vi "Autonomous.vi"() -> ()   [LabVIEW 2019]
doc: "This VI starts when autonomous period begins, and will automatically be terminated when it ends. You can carry out timed or sensor driven operations directly to I/O or to subsystems without needing to return to the caller."
uses:
  <vilib>/Rock Robotics/WPI/Utilities/WPI_GetSetVariantRefNum.vi
  <vilib>/Rock Robotics/Network Tables/NT Read String.vi
panel:
  in  "goto":string
  in  "start":string
  in  "milliseconds to wait":u32
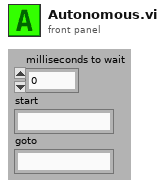
[diagram p1: front panel]
types:
  T1 = typedef "WPI_JoystickDevRef.ctl" = cluster{"Device":T2}
  T2 = typedef "WPI_JoystickDeviceEnum.ctl" = enum16{"USB 0", "USB 1", "USB 2", "USB 3", "USB 4", "USB 5"}
  T3 = typedef "Command Status Info.ctl" = cluster{"Name":string, "Status":T4, "notifier out":T5}
  T4 = typedef "Completion Status.ctl" = enum16{"Successful", "Aborted", "Incomplete"}
  T5 = typedef "Completion Notifier.ctl" = refnum<notifier>
  T6 = typedef "WPI_MotorControlDeviceRef.ctl" = cluster{"DeviceStatus":errorcluster, "Type":T7, "PWM":cluster{"PWM Channel":T8, "DeadBand":T9}, "CAN":cluster{"Device Number":u8, "SetOutput VI Ref":variant, "GetOutput VI Ref":variant, "Enable VI Ref":variant, "Disable VI Ref":variant, "Data":variant}, "Invert":bool, "DIO PWM":cluster{"PWM \"Enable\" Channel":T8, "DIOChannel":T10, "PWM Rate":dbl}}
  T7 = typedef "WPI_MotorControlType.ctl" = enum16{"PWM", "CAN", "DIO PWM"}
  T8 = typedef "FPGA_DIOPWMChannel.ctl" = enum8{"PWM 0", "PWM 1", "PWM 2", "PWM 3", "PWM 4", "PWM 5", "PWM 6", "PWM 7", "PWM 8", "PWM 9", "PWM MXP 0", "PWM MXP 1", "PWM MXP 2", "PWM MXP 3", "PWM MXP 4", "PWM MXP 5", "PWM MXP 6", "PWM MXP 7", "PWM MXP 8", "PWM MXP 9", "Invalid"}
  T9 = typedef "WPI_PWMDeadband.ctl" = cluster{"Name":string, "maxPositivePwm":i32, "minPositivePwm":i32, "centerPwm":i32, "maxNegativePwm":i32, "minNegativePwm":i32, "angularRange":u16}
  T10 = typedef "FPGA_DIOChannel.ctl" = enum8{"DIO 0", "DIO 1", "DIO 2", "DIO 3", "DIO 4", "DIO 5", "DIO 6", "DIO 7", "DIO 8", "DIO 9", "DIO MXP 0", "DIO MXP 1", "DIO MXP 2", "DIO MXP 3", "DIO MXP 4", "DIO MXP 5", "DIO MXP 6", "DIO MXP 7", "DIO MXP 8", "DIO MXP 9", "DIO MXP 10", "DIO MXP 11", "DIO MXP 12", "DIO MXP 13", "DIO MXP 14", "DIO MXP 15", "SPI Port CS1", "SPI Port CS2", "SPI Port CS3", "SPI Port MISO", "SPI Port MOSI", "Invalid"}
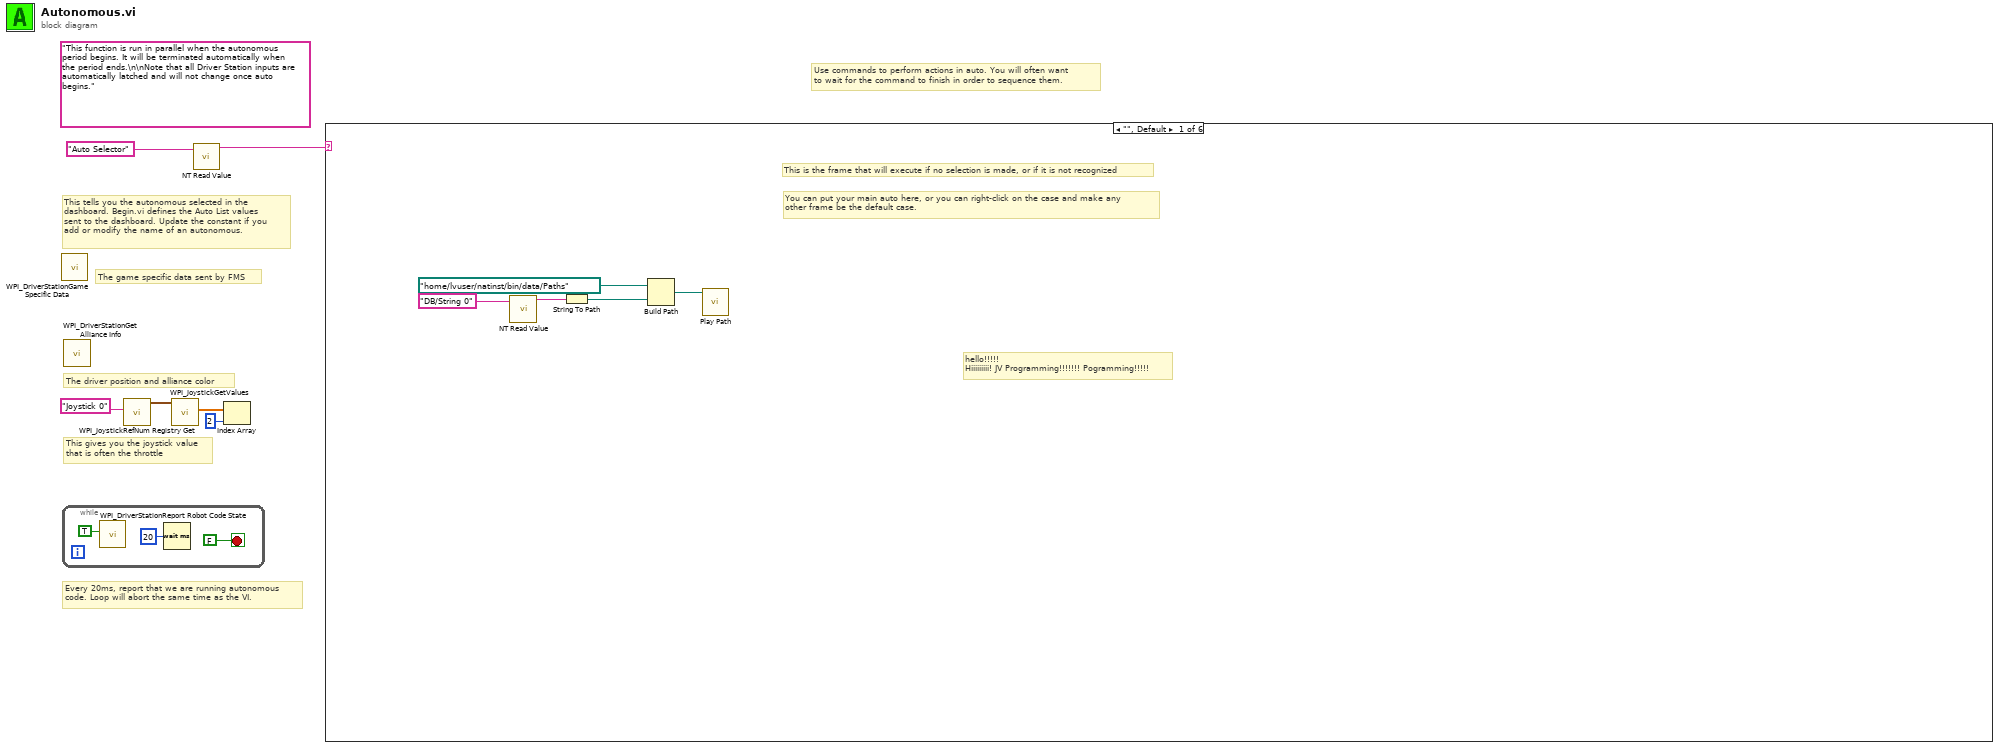
[diagram p0: block diagram]
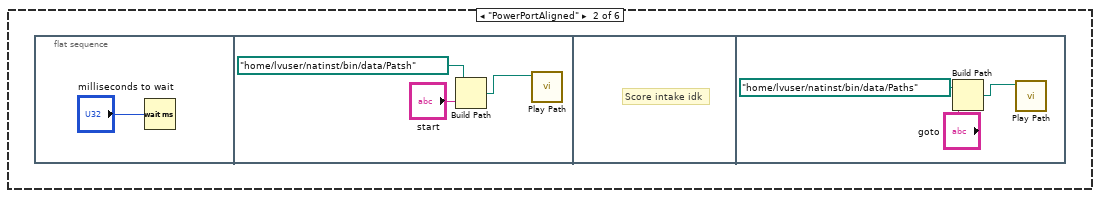
[diagram p2: hidden frame]
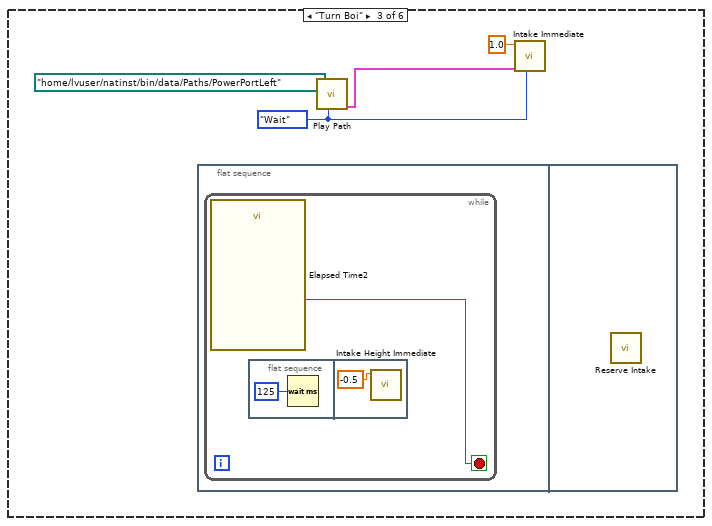
[diagram p3: hidden frame]
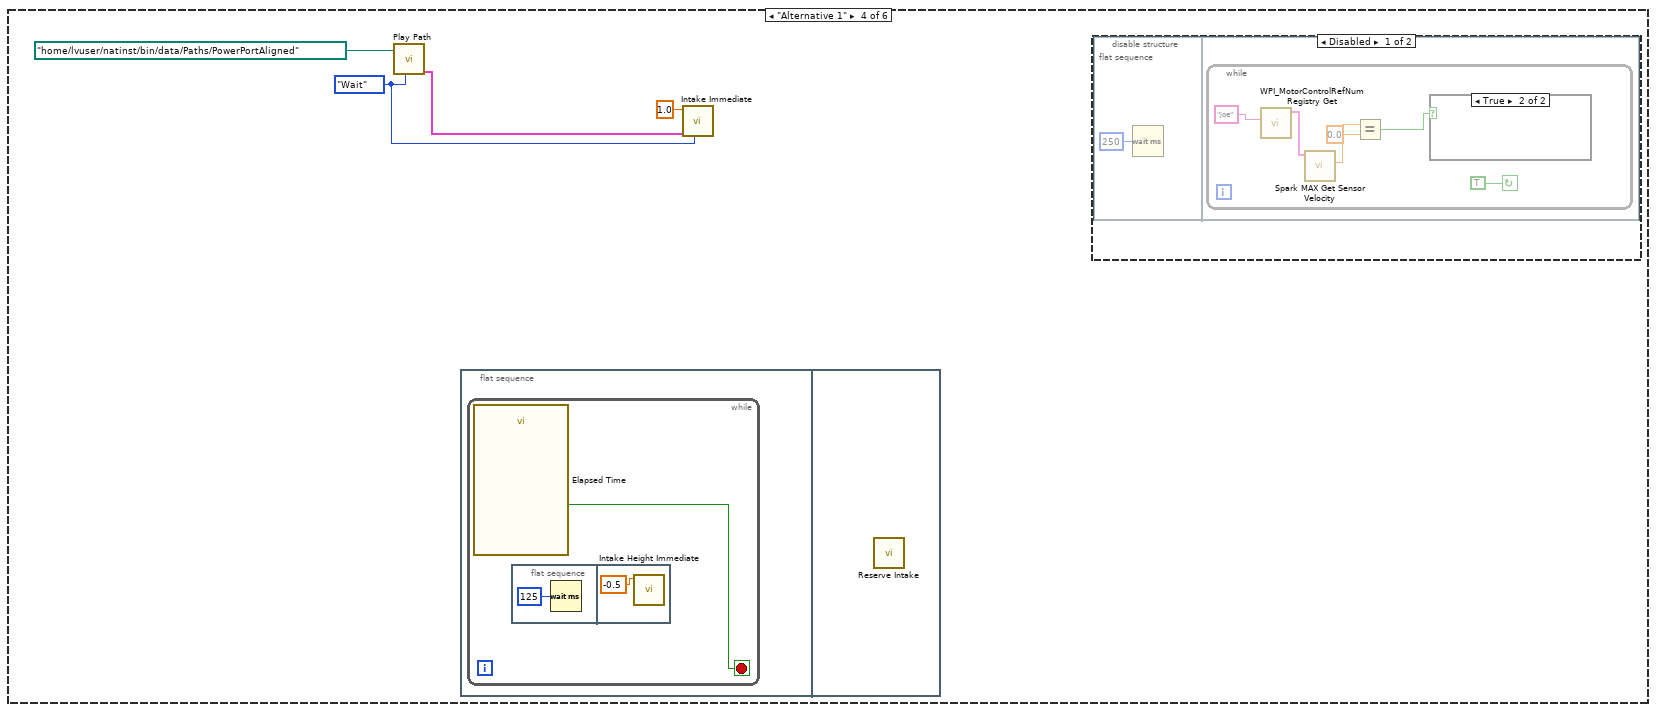
[diagram p4: hidden frame]
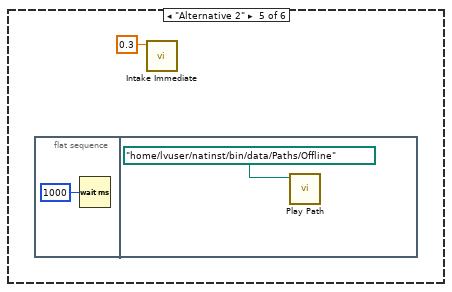
[diagram p7: hidden frame]
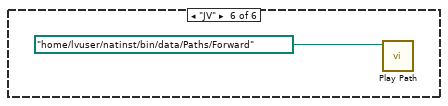
[diagram p8: hidden frame]
diagram:
  (unwired) "This function is run in parallel when the autonomous period begins. It will be terminated automatically when the period ends.\n\nNote that all Driver Station inputs are automatically latched and will not change once auto begins."
  # "The game specific data sent by FMS"
  # "This tells you the autonomous selected in the \ndashboard. Begin.vi defines the Auto List values\nsent to the dashboard. Update the constant if you\nadd or modify the name of an autonomous."
  # "Every 20ms, report that we are running autonomous\ncode. Loop will abort the same time as the VI."
  # "This gives you the joystick value\nthat is often the throttle"
  # "Use commands to perform actions in auto. You will often want\nto wait for the command to finish in order to sequence them."
  # "The driver position and alliance color"
  n1 = call <vilib>:"WPI_DriverStationGame Specific Data.vi"() -> ()  [unwired: 11 in, 1 out]
  n2 = while {
    stop <- FALSE stop-if-true
    n3 = call <vilib>:"WPI_DriverStationReport Robot Code State.vi"("Autonomous"=TRUE) -> ()  [unwired: 10 in, 1 out]
    n4 = Wait (ms)(milliseconds to wait=u32 20) -> ()  [unwired: 1 out]
  }
  n5 = call <vilib>:"WPI_DriverStationGet Alliance Info.vi"() -> ()  [unwired: 12 out]
  n6 = call <vilib>:"WPI_JoystickRefNum Registry Get.vi"("refnum name"="Joystick 0") -> ("JoystickDevRef"=w5:T1)  [unwired: 1 in, 9 out]
  n7 = call <vilib>:"WPI_JoystickGetValues.vi"("JoystickDevRef"=w5) -> ("Axes"=w4:dbl[])  [unwired: 6 in, 4 out]
  n8 = call-poly <vilib>:"NT Read Value.vi"("Name"="Auto Selector") -> ("String"=w1:string)  [unwired: 9 in, 1 out]
  n9 = Index Array(array=w4, index=2) -> ()  [unwired: 1 out]
  n10 = case shown="\"\", Default" w1 {
    frame "", Default {
      # "hello!!!!!\nHiiiiiiiii! JV Programming!!!!!!! Pogramming!!!!!"
      # "You can put your main auto here, or you can right-click on the case and make any\nother frame be the default case."
      # "This is the frame that will execute if no selection is made, or if it is not recognized"
      n11 = call-poly <vilib>:"NT Read Value.vi"("Name"="DB/String 0") -> ("String"=w11:string)  [unwired: 9 in, 1 out]
      n12 = String To Path(string=w11) -> (path=w10:path)
      n13 = Build Path(base path=path "/home/lvuser/natinst/bin/data/Paths" ("Path"), name or relative path=w10) -> (appended path=w13:path)
      n14 = call "Play Path.vi"("Path"=w13) -> ()  [unwired: 10 in, 1 out]
    }
    frame "PowerPortAligned" {
      n15 = flat-sequence {
        frame #0 {
          n16 = Wait (ms)(milliseconds to wait="milliseconds to wait") -> ()  [unwired: 1 out]
        }
        frame #1 {
          n17 = Build Path(base path=path "/home/lvuser/natinst/bin/data/Patsh", name or relative path="start") -> (appended path=w16:path)
          n18 = call "Play Path.vi"("Path"=w16) -> ()  [unwired: 10 in, 1 out]
        }
        frame #2 {
          # "Score intake idk"
        }
        frame #3 {
          n19 = Build Path(base path=path "/home/lvuser/natinst/bin/data/Paths", name or relative path="goto") -> (appended path=w21:path)
          n20 = call "Play Path.vi"("Path"=w21) -> ()  [unwired: 10 in, 1 out]
        }
      }
    }
    frame "Turn Boi" {
      w22 = enum16{"Start", "Wait"}."Wait" ("Synchronication")
      n21 = flat-sequence {
        frame #0 {
          n22 = while {
            stop <- w26 stop-if-true
            n23 = call "Elapsed Time2"() -> ("Time has Elapsed"=w26:bool)  [unwired: 12 in, 7 out]
            n24 = flat-sequence {
              frame #0 {
                n25 = Wait (ms)(milliseconds to wait=u32 125) -> ()  [unwired: 1 out]
              }
              frame #1 {
                n26 = call "Intake Height Immediate.vi"("Setpoint"=-0.5) -> ()  [unwired: 10 in, 1 out]
              }
            }
          }
        }
        frame #1 {
          n27 = call "Reserve Intake.vi"() -> ()  [unwired: 11 in, 1 out]
        }
      }
      n28 = call "Play Path.vi"("Synchronication"=w22, "Path"=path "/home/lvuser/natinst/bin/data/Paths/PowerPortLeft") -> ("Command Info Out"=w23:T3)  [unwired: 9 in]
      n29 = call "Intake Immediate.vi"("Synchronication"=w22, "Command Info In"=w23, "Setpoint"=1.0) -> ()  [unwired: 8 in, 1 out]
    }
    frame "Alternative 1" {
      w30 = enum16{"Start", "Wait"}."Wait" ("Synchronication")
      n30 = call "Play Path.vi"("Synchronication"=w30, "Path"=path "/home/lvuser/natinst/bin/data/Paths/PowerPortAligned") -> ("Command Info Out"=w31:T3)  [unwired: 9 in]
      n31 = flat-sequence {
        frame #0 {
          n32 = while {
            stop <- w33 stop-if-true
            n33 = call "Elapsed Time"() -> ("Time has Elapsed"=w33:bool)  [unwired: 12 in, 7 out]
            n34 = flat-sequence {
              frame #0 {
                n35 = Wait (ms)(milliseconds to wait=u32 125) -> ()  [unwired: 1 out]
              }
              frame #1 {
                n36 = call "Intake Height Immediate.vi"("Setpoint"=-0.5) -> ()  [unwired: 10 in, 1 out]
              }
            }
          }
        }
        frame #1 {
          n37 = call "Reserve Intake.vi"() -> ()  [unwired: 11 in, 1 out]
        }
      }
      n38 = call "Intake Immediate.vi"("Synchronication"=w30, "Command Info In"=w31, "Setpoint"=1.0) -> ()  [unwired: 8 in, 1 out]
      n39 = disable-structure shown="Disabled" {
        frame Disabled {
          n40 = flat-sequence {
            frame #0 {
              n41 = Wait (ms)(milliseconds to wait=u32 250) -> ()  [unwired: 1 out]
            }
            frame #1 {
              n42 = while {
                stop <- TRUE continue-if-true
                n43 = call <vilib>:"WPI_MotorControlRefNum Registry Get.vi"("refnum name"="joe") -> ("MotorControlDevRef"=w40:T6)  [unwired: 9 in, 1 out]
                n44 = call <vilib>:"Spark MAX Get Sensor Velocity.vi"("MotorControlDevRef in"=w40) -> ("Sensor Velocity"=w39:dbl)  [unwired: 7 in, 3 out]
                n45 = Equal?(x=w39, y=0.0) -> (x = y?=w37:bool)
                n46 = case shown="True" w37 {
                  frame False {
                  }
                  frame True {
                  }
                }
              }
            }
          }
        }
        frame Enabled {
        }
      }
    }
    frame "Alternative 2" {
      n47 = flat-sequence {
        frame #0 {
          n48 = Wait (ms)(milliseconds to wait=u32 1000) -> ()  [unwired: 1 out]
        }
        frame #1 {
          n49 = call "Play Path.vi"("Path"=path "/home/lvuser/natinst/bin/data/Paths/Offline") -> ()  [unwired: 10 in, 1 out]
        }
      }
      n50 = call "Intake Immediate.vi"("Setpoint"=0.3) -> ()  [unwired: 10 in, 1 out]
    }
    frame "JV" {
      n51 = call "Play Path.vi"("Path"=path "/home/lvuser/natinst/bin/data/Paths/Forward") -> ()  [unwired: 10 in, 1 out]
    }
  }
